vi "Script from Excel.vi"() -> ()   [LabVIEW 2019, in "Simple SysDef API.lvlib"]
uses:
  <userlib>/SimpleSysDef/Simple SysDef API.lvlib
  <userlib>/SimpleSysDef/_SubVIs/Add Target_Settings.ctl
  <userlib>/SimpleSysDef/_SubVIs/Add Target_Types.ctl
  <userlib>/SimpleSysDef/_SubVIs/Create New System Definition.vi
  <userlib>/SimpleSysDef/_SubVIs/Add Target.vi
  <userlib>/SimpleSysDef/_SubVIs/Save and Close System Definition.vi
panel:
  out "SysDef Path":path
  out "error out":errorcluster
  in  "error in (no error)":errorcluster
  in  "Configuration Path":path=path "C:/Addons/Simple-System-Definition-API/Source/Examples/_Files/SampleConfiguration.xlsx"
  in  "Sysdef Name":string="ExcelConvert.nivssdf"
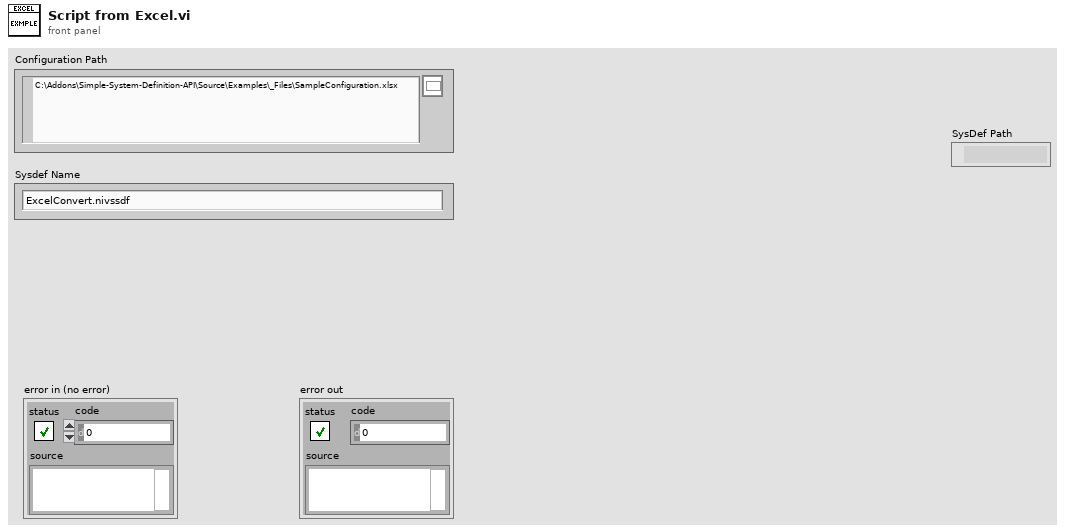
[diagram p1: front panel]
types:
  T1 = typedef "Simple SysDef API.lvlib/Add Target_Settings.ctl" = cluster{"Name":string, "Target Type":T2, "IPAddress":string, "PrimaryControlLoopProcessor":i32, "DataProcessingLoopProcessor":i32, "DataProcessingLoopDecimation":i32, "DAQDigitalLinesDecimation":u32, "MaximumStreamedChannels":i32, "ExecutionMode":i32, "FilterDAQErrors":bool, "FilterWatchdogErrors":bool, "FPGAScanInterfaceMode":u16, "TargetRate":dbl}
  T2 = typedef "Simple SysDef API.lvlib/Add Target_Types.ctl" = string
  T3 = typedef "Simple SysDef API.lvlib/Edit Chassis_Settings.ctl" = cluster{"Name":string, "Master Chassis":T4}
  T4 = typedef "Simple SysDef API.lvlib/Add Chassis_DAQ Master Settings.ctl" = cluster{"Type":T5, "DAQ Name":string, "clkSrc":i32, "activeEdge":i32, "exportClk":i32, "exportClkToLine":i32, "triggerLine":i32, "triggerSlope":i32, "startTrigger":i32, "startTriggerLine":i32}
  T5 = typedef "Simple SysDef API.lvlib/Add Chassis_Type.ctl" = enum16{"None", "DAQ", "FPGA", "Timing and Sync", "Automatic"}
  T6 = typedef "Simple SysDef API.lvlib/Add DAQ Hardware_Settings.ctl" = cluster{"Name":string, "Description":string, "InputConfiguration":i32, "TurnOffHWTimedSinglePointAI":bool, "TurnOffHWTimedSinglePointAO":bool, "DAQConversionRateOption":i32, "PortWidth":u16, "Analog Inputs":T7[], "Analog Outputs":T7[], "DIO Port Settings":T8[], "Counter Settings":cluster{"Frequency Measurements":T10[], "Period Measurements":T10[], "Count Measurements":T11[], "Position Measurements":T12[]}}
  T7 = typedef "Simple SysDef API.lvlib/Add DAQ Hardware_Analog Settings.ctl" = cluster{"Name":string, "Units":string, "InitialValue":dbl, "HighLevel":dbl, "LowLevel":dbl, "Channel":u32, "ChannelType":i32, "Alias Name":string}
  T8 = typedef "Simple SysDef API.lvlib/Add DAQ Hardware_Digital Port Settings.ctl" = cluster{"portNumber":u32, "Inverted":bool, "Digital Inputs":T9[], "Digital Outputs":T9[]}
  T9 = typedef "Simple SysDef API.lvlib/Add DAQ Hardware_Digital Settings.ctl" = cluster{"Name":string, "InitialValue":bool, "DigitalLine":u32, "Alias Name":string}
  T10 = typedef "Simple SysDef API.lvlib/Add Frequency Measurement Channels_Settings.ctl" = cluster{"Name":string, "Description":string, "Units":string, "Counter":u32, "DefaultValue":dbl, "Maximum":dbl, "Minimum":dbl, "Edge":i32, "Alias Name":string}
  T11 = typedef "Simple SysDef API.lvlib/Add Count Measurement Channels_Settings.ctl" = cluster{"Name":string, "Description":string, "Units":string, "Counter":u32, "DefaultValue":dbl, "CountDirection":i32, "Edge":i32, "ResetVariable":refnum<k24>, "Alias Name":string}
  T12 = typedef "Simple SysDef API.lvlib/Add Position Measurement Channels_Settings.ctl" = cluster{"Name":string, "Description":string, "Units":string, "Counter":u32, "DefaultValue":dbl, "Decoding":i32, "ZIndexMode":i32, "Alias Name":string}
  T13 = typedef "Simple SysDef API.lvlib/Add FPGA Hardware_Settings.ctl" = cluster{"Path":path, "RIO Name":string, "Aliases":cluster{"Relative Node Path":string, "Alias Name":string}[]}
  T14 = typedef "Simple SysDef API.lvlib/Add NI-XNET CAN Hardware_Port Settings.ctl" = cluster{"Name":string, "Database Name":string, "PortNumber":u16, "ClusterName":string, "BaudRate":u32, "InlineIncoming":bool, "IncomingRate":u32, "InlineOutgoing":bool, "OutgoingRate":u32, "Termination":i32, "Echo":bool, "InputStreamQueueSize":u32, "CANBusOff":bool, "CANBusOffRate":u32, "TransceiverType":i32, "TransmitOrderType":i32, "Cyclic Frames":T15[], "Outgoing Frames":T18[], "Incoming Frames":T16[], "Log Files":T19[]}
  T15 = typedef "Simple SysDef API.lvlib/Add NI-XNET CAN Hardware_Periodic Frame Settings.ctl" = cluster{"Frame Settings":T16, "Trigger Node Path":string, "TriggerType":i32, "Disable Node Path":string}
  T16 = typedef "Simple SysDef API.lvlib/Add NI-XNET CAN Hardware_Frame Settings.ctl" = cluster{"Name":string, "ID":u32, "PayloadLength":u32, "StartTimeOffset":dbl, "Enable64Bit":bool, "Signals":T17[]}
  T17 = typedef "Simple SysDef API.lvlib/Add NI-XNET CAN Hardware_Signal Settings.ctl" = cluster{"Name":string, "Description":string, "Units":string, "DefaultValue":dbl, "Alias Name":string}
  T18 = typedef "Simple SysDef API.lvlib/Add NI-XNET CAN Hardware_Sporadic Frame Settings.ctl" = cluster{"Frame Settings":T16, "Trigger Node Path":string, "TriggerType":i32, "Disable Node Path":string, "EnableSoftwareCyclicTrigger":bool, "TransmitTime":dbl, "Phase":i32}
  T19 = typedef "Simple SysDef API.lvlib/Add NI-XNET CAN Hardware_Add Log File_Settings.ctl" = cluster{"Name":string, "Filename":string, "Destination Folder":path, "NumberOfBytesToRead":u32, "DataLoggingFileType":i32, "TDMSGroupName":string, "TDMSChannelName":string, "Filter":i32, "FrameIDs":string[], "TriggerType":i32, "LimitType":i32, "LimitValue":u32, "Operation":i32, "Retriggerable":bool, "Trigger Node Path":string}
  T20 = cluster{"Chassis Settings":T3, "DAQ Boards":T6[], "FPGA Boards":T13[], "CAN Boards":T14[]}
  T21 = typedef "Simple SysDef API.lvlib/System Definition Reference.ctl" = refnum<k24>
  T22 = typedef "Simple SysDef API.lvlib/Target Node Paths.ctl" = cluster{"Hardware":string, "Custom Devices":string, "Simulation Models":string, "User Channels":string, "Calculated Channels":string, "Stimulus":string, "Alarms":string, "Procedures":string}
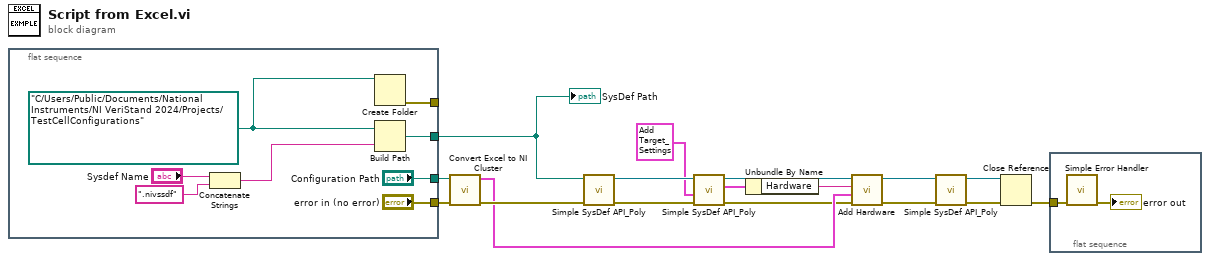
[diagram p0: block diagram]
diagram:
  n1 = flat-sequence {
    tunnel: ["error in (no error)"] -> w17
    tunnel: ["Configuration Path"] -> w16
    tunnel: [w18] -> w14
    tunnel: [w23] -> _
    frame #0 {
      w19 = path "C:/Users/Public/Documents/National Instruments/NI VeriStand 2024/Projects/TestCellConfigurations"
      n2 = Concatenate Strings("Sysdef Name", ".nivssdf" ("string")) -> (w21:string)
      n3 = Create Folder(path (use dialog)=w19) -> (error out=w23:errorcluster)  [unwired: 2 in, 2 out]
      n4 = Build Path(base path=w19, name or relative path=w21) -> (appended path=w18:path)
    }
  }
  n5 = call <userlib>:"Convert Excel to NI Cluster.vi"("error in"=w17, "path"=w16) -> ("error out"=w15:errorcluster, "Chassis Settings"=w6:T20)  [unwired: 8 in]
  n6 = call-poly <userlib>:"Simple SysDef API_Poly.vi"("error in (no error)"=w15, "path"=w14) -> ("error out"=w12:errorcluster, "SysDef Ref"=w13:T21)  [unwired: 7 in, 1 out]
  n7 = call-poly <userlib>:"Simple SysDef API_Poly.vi"("error in (no error)"=w12, "Settings"=T1 {"Name"="Controller", "Target Type"="PharLap", "IPAddress"="192.168.1.1", "PrimaryControlLoopProcessor"=-2, "DataProcessingLoopProcessor"=-2, "DataProcessingLoopDecimation"=1, "DAQDigitalLinesDecimation"=1, "MaximumStreamedChannels"=512, "ExecutionMode"=0, "FilterDAQErrors"=FALSE, "FilterWatchdogErrors"=FALSE, "FPGAScanInterfaceMode"=0, "TargetRate"=100.0}, "SysDef Ref"=w13) -> ("error out"=w5:errorcluster, "Target Node Paths"=w10:T22, "SysDef Ref Out"=w3:T21)  [unwired: 6 in]
  n8 = Unbundle By Name(w10) -> ("Hardware"=w4:string)
  n9 = call <userlib>:"Add Hardware.vi"("error in (no error)"=w5, "Chassis Settings"=w6, "Hardware"=w4, "System Definition Ref"=w3) -> ("error out"=w2:errorcluster, "System Definition Ref"=w1:T21)  [unwired: 6 in]
  n10 = call-poly <userlib>:"Simple SysDef API_Poly.vi"("error in (no error)"=w2, "SysDef Ref"=w1) -> ("error out"=w9:errorcluster, "SysDef Ref out"=w8:T21)  [unwired: 8 in]
  n11 = Close Reference(reference=w8, error in (no error)=w9) -> (error out=w7:errorcluster)
  n12 = flat-sequence {
    tunnel: w7 -> [w27]
    frame #0 {
      n13 = call <vilib>:"Simple Error Handler.vi"("error in (no error)"=w27) -> ("error out"=→"error out":errorcluster)  [unwired: 4 in, 4 out]
    }
  }
  "SysDef Path" <- w14
